vi "SSI PR Pump Test.vi"() -> ()   [LabVIEW 2018, in "SSI PR Pump.lvlib"]
uses:
  SSI PR Pump.lvlib
  SSI PR Settings Cluster.ctl
panel:
  out "Pressure":dbl format="%#_13g"
  in  "speed (ml/min)":dbl min=0.0 max=999.99 format="%06.2f"
  in  "?":bool
  out "Pump On?":enum16{"Off", "On", "Not Initialized"}(ring)
  out "Flow":dbl
  out "Connection Error":bool
  in  "Pause":bool
  out "Initialized":bool
  out "No Pump Connected":bool
  out "error out":errorcluster
  in  "error in (no error)":errorcluster
  out "SSI PR Settings Out":T1={"VISA resource name"="", "Simulated?"=TRUE}
  in  "SSI PR Settings In":T1
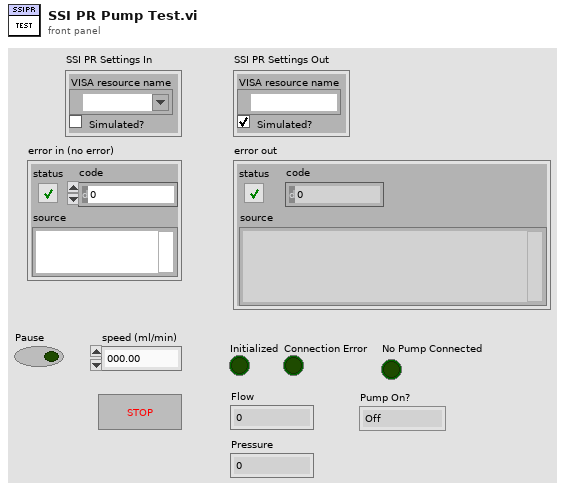
[diagram p1: front panel]
types:
  T1 = typedef "SSI PR Pump.lvlib/SSI PR Settings Cluster.ctl" = cluster{"VISA resource name":refnum<visa-resource-name>, "Simulated?":bool}
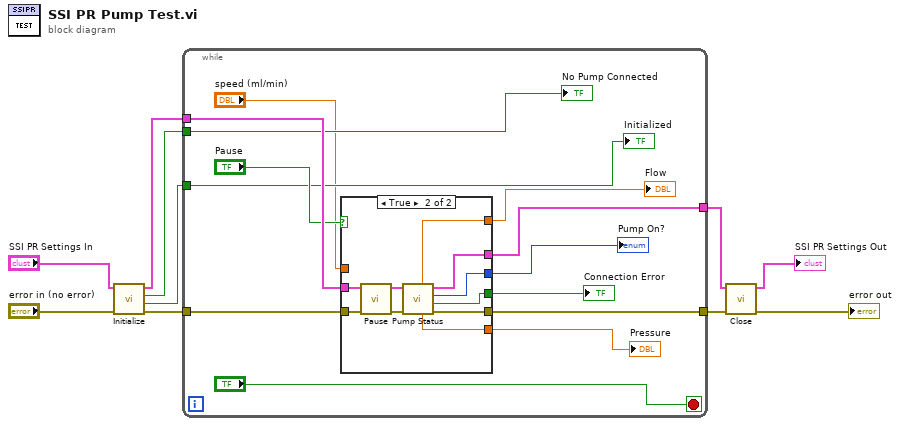
[diagram p0: block diagram]
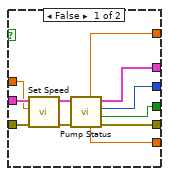
[diagram p2: hidden frame]
diagram:
  n1 = call "Initialize.vi"("error in (no error)"="error in (no error)", "SSI PR Settings In"="SSI PR Settings In") -> ("error out"=w1:errorcluster, "Initialized"=w5:bool, "No Pump Connected"=w6:bool, "SSI PR Settings Out"=w3:T1)  [unwired: 6 in]
  n2 = while {
    tunnel: w6 -> [w17]
    tunnel: w5 -> [w18]
    tunnel: [w23] -> w4
    tunnel: w3 -> [w22]
    tunnel: [w21] -> w2
    tunnel: w1 -> [w20]
    stop <- "?" stop-if-true
    n3 = case shown="True" "Pause" {
      tunnel: [w30 w39] -> w23
      tunnel: w22 -> [w34 w44]
      tunnel: [w29 w40] -> w21
      tunnel: w20 -> [w33 w43]
      tunnel: [w28 w38] -> w15
      tunnel: [w25 w36] -> w14
      tunnel: [w27 w37] -> w16
      tunnel: "speed (ml/min)" -> [w26 _]
      tunnel: [w24 w35] -> w11
      frame False {
        n4 = call "Set Speed.vi"("error in (no error)"=w33, "speed (ml/min)"=w26, "SSI PR Settings"=w34) -> ("error out"=w31:errorcluster, "SSI PR Settings"=w32:T1)  [unwired: 6 in, 1 out]
        n5 = call "Pump Status.vi"("error in (no error)"=w31, "SSI PR Settings"=w32) -> ("error out"=w29:errorcluster, "Connection Error"=w28:bool, "Pump On?"=w27:enum16{"Off", "On", "Not Initialized"}, "SSI PR Settings"=w30:T1, "Pressure"=w24:dbl, "Flow"=w25:dbl)  [unwired: 4 in]
      }
      frame True {
        n6 = call "Pause.vi"("error in (no error)"=w43, "SSI PR Settings"=w44) -> ("error out"=w41:errorcluster, "SSI PR Settings"=w42:T1)  [unwired: 6 in, 1 out]
        n7 = call "Pump Status.vi"("error in (no error)"=w41, "SSI PR Settings"=w42) -> ("error out"=w40:errorcluster, "Connection Error"=w38:bool, "Pump On?"=w37:enum16{"Off", "On", "Not Initialized"}, "SSI PR Settings"=w39:T1, "Pressure"=w35:dbl, "Flow"=w36:dbl)  [unwired: 4 in]
      }
    }
    "Connection Error" <- w15
    "Pump On?" <- w16
    "Flow" <- w14
    "Pressure" <- w11
    "No Pump Connected" <- w17
    "Initialized" <- w18
  }
  n8 = call "Close.vi"("error in (no error)"=w2, "SSI PR Settings In"=w4) -> ("error out"=→"error out":errorcluster, "SSI PR Settings Out"=→"SSI PR Settings Out":T1)  [unwired: 7 in, 1 out]
